vi "cno_generate scaling vector.vi"(7 "cno data":T1, 10 "P":dbl[](array[numeric]), 11 "OB":dbl[](array[numeric])) -> (3 "scaling vector":dbl[](array[numeric]))   [LabVIEW 2020, in "NI_Gmath.lvlib"]
uses:
  NI_Gmath.lvlib
  cno_data.ctl
  ones_1d.vi
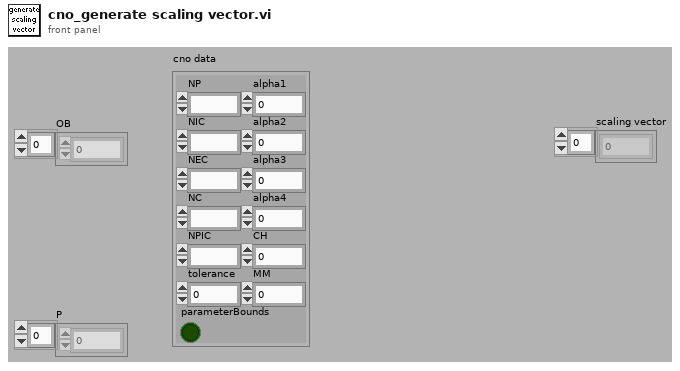
[diagram p1: front panel]
types:
  T1 = typedef "NI_Gmath.lvlib/cno_data.ctl" = cluster{"NP":i32, "NIC":i32, "NEC":i32, "NC":i32, "NPIC":i32, "parameterBounds":bool, "alpha1":dbl, "alpha2":dbl, "alpha3":dbl, "alpha4":dbl, "CH":i32, "MM":i32, "tolerance":dbl}
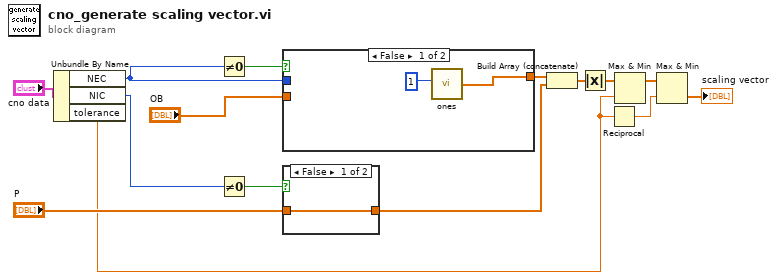
[diagram p0: block diagram]
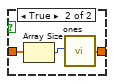
[diagram p2: hidden frame]
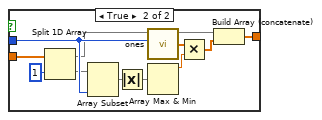
[diagram p3: hidden frame]
diagram:
  n1 = Unbundle By Name("cno data") -> ("NEC"=w3:i32, "NIC"=w2:i32, "tolerance"=w1:dbl)
  n2 = Not Equal To 0?(x=w3) -> (x != 0?=w5:bool)
  n3 = Not Equal To 0?(x=w2) -> (x != 0?=w6:bool)
  n4 = case shown="False" w5 {
    tunnel: "OB" -> [_ w25]
    tunnel: w3 -> [_ w28]
    tunnel: [w16 w18] -> w10
    frame False {
      n5 = call-poly "ones.vi"("m"=1) -> ("ones"=w16:dbl[])  [unwired: 7 in]
    }
    frame True {
      n6 = Split 1D Array(array=w25, index=1) -> (first subarray=w24:dbl[], second subarray=w27:dbl[])
      n7 = Array Subset(array=w27, length=w28) -> (w23:dbl[])  [unwired: 1 in]
      n8 = Absolute Value(x=w23) -> (abs(x)=w22:dbl[])
      n9 = call-poly "ones.vi"("m"=w28) -> ("ones"=w21:dbl[])  [unwired: 7 in]
      n10 = Array Max & Min(array=w22) -> (max value=w20:dbl)  [unwired: 3 out]
      n11 = Multiply(x=w21, y=w20) -> (x*y=w19:dbl[])
      n12 = Build Array (concatenate)(w24, w19) -> (w18:dbl[])
    }
  }
  n13 = case shown="False" w6 {
    tunnel: "P" -> [w29 w32]
    tunnel: [w29 w30] -> w11
    frame False {
    }
    frame True {
      n14 = Array Size(array=w32) -> (size(s)=w31:i32)
      n15 = call-poly "ones.vi"("m"=w31) -> ("ones"=w30:dbl[])  [unwired: 7 in]
    }
  }
  n16 = Build Array (concatenate)(w10, w11) -> (w12:dbl[])
  n17 = Absolute Value(x=w12) -> (abs(x)=w7:dbl[])
  n18 = Reciprocal(x=w1) -> (1/x=w9:dbl)
  n19 = Max & Min(x=w7, y=w1) -> (max(x,y)=w8:dbl[])  [unwired: 1 out]
  n20 = Max & Min(x=w8, y=w9) -> (min(x,y)=→"scaling vector":dbl[])  [unwired: 1 out]
